vi "Gas Flow 2.vi"() -> ()   [LabVIEW 2011]
uses:
  GlobalVariables.vi
panel:
  out "TMGa #2 2":string="TMGa #2"
  out "MFC Left 8":string="TMIn #1"
  out "MFC Left 7":string="TMIn #1"
  out "MFC Left 6":string="TMIn #1"
  out "MFC Left 5":string="TMIn #1"
  out "MFC Left 4":string="TMIn #1"
  out "MFC Left 3":string="TMIn #1"
  out "MFC Left 2":string="TMIn #1"
  out "MFC Left":string="TMIn #1"
  out "DMHy":string="DMHy"
  out "TMAl #2":string="TMAl #2"
  out "TMAl #1":string="TMAl #1"
  out "TMGa #2":string="TMGa #2"
  out "TMGa #1":string="TMGa #1"
  out "TMIn #2":string="TMIn #2"
  out "Spare":string="Spare"
  out "TMIn #1":string="TMIn #1"
  out "CCl4":string="CCl4"
  out "DEZn":string="DEZn"
  in  "19":bool caption="49"
  in  "20":bool caption="49"
  in  "29":bool caption="49"
  in  "53":bool caption="49"
  in  "54":bool caption="49"
  in  "55":bool caption="49"
  in  "77":bool caption="49"
  in  "78":bool caption="49"
  in  "79":bool caption="49"
  in  "80":bool caption="49"
  in  "56":bool caption="49"
  in  "81":bool caption="49"
  in  "84":bool caption="49"
  in  "24":bool caption="49"
  in  "24":bool caption="49"
  in  "Flip 91/92":bool
  in  "MFC 55":dbl
  out "MFC 54":dbl
  in  "MFC 53":dbl
  out "MFC 52":dbl
  in  "Flip 33/34":bool
  in  "MFC 51":dbl
  out "MFC 50":dbl
  in  "23":bool caption="49"
  in  "25":bool caption="49"
  in  "MFC 49":dbl
  out "MFC 48":dbl
  in  "26":bool caption="49"
  in  "76":bool caption="49"
  in  "75":bool caption="49"
  in  "66":bool caption="49"
  in  "65":bool caption="49"
  in  "68":bool caption="49"
  in  "67":bool caption="49"
  in  "70":bool caption="49"
  in  "69":bool caption="49"
  in  "72":bool caption="49"
  in  "71":bool caption="49"
  in  "74":bool caption="49"
  in  "73":bool caption="49"
  in  "52":bool caption="49"
  in  "51":bool caption="49"
  in  "34":bool caption="49"
  in  "33":bool caption="49"
  in  "MFC10":dbl
  in  "MFC 45":dbl
  in  "MFC 44":dbl
  in  "MFC 01":dbl
  out "MFC10":dbl
  out "MFC 45":dbl
  out "MFC 44":dbl
  out "MFC 01":dbl
  in  "22":bool caption="49"
  in  "21":bool caption="49"
  in  "22":bool caption="49"
  in  "01":bool caption="49"
  in  "02":bool caption="49"
  in  "02":bool caption="49"
  in  "59":bool caption="49"
  in  "27":bool caption="49"
  in  "30":bool caption="49"
  in  "94":bool caption="49"
  in  "93":bool caption="49"
  in  "?":bool caption="49"
  in  "28":bool caption="49"
  in  "31":bool caption="49"
  in  "95":bool caption="49"
  in  "96":bool caption="49"
  in  "90":bool caption="49"
  in  "92":bool caption="49"
  in  "91":bool caption="49"
  in  "CloseVi?":bool
  in  "Close":bool
  # "19"
  # "20"
  # "71/72"
  # "TO EBARA"
  # "Arsine"
  # "AsH3 1-DD VENT"
  # "32"
  # "21"
  # "H2"
  # "33"
  # "TO TURBO PUMP"
  # "23"
  # "69/70"
  # "22"
  # "AsH3 2-DD VENT"
  # "24"
  # "Si2H6 DD VENT"
  # "34"
  # "67/68"
  # "HYDRIDE GROWTH"
  # "Phosphine"
  # "35"
  # "38"
  # "42"
  # "Si2H6 DD VENT"
  # "HYDRIDE VENT"
  # "?"
  # "36"
  # "TO SHROUD"
  # "39"
  # "TO PURGE"
  # "41"
  # "N2"
  # "41"
  # "57"
  # "TO GLOVE BOX"
  # "28"
  # "ALKYL GROWTH"
  # "ALKYL VENT"
  # "27"
  # "ALKYL DD VENT"
  # "57"
  # "28"
  # "27"
  # "VACUUM"
  # "VENT"
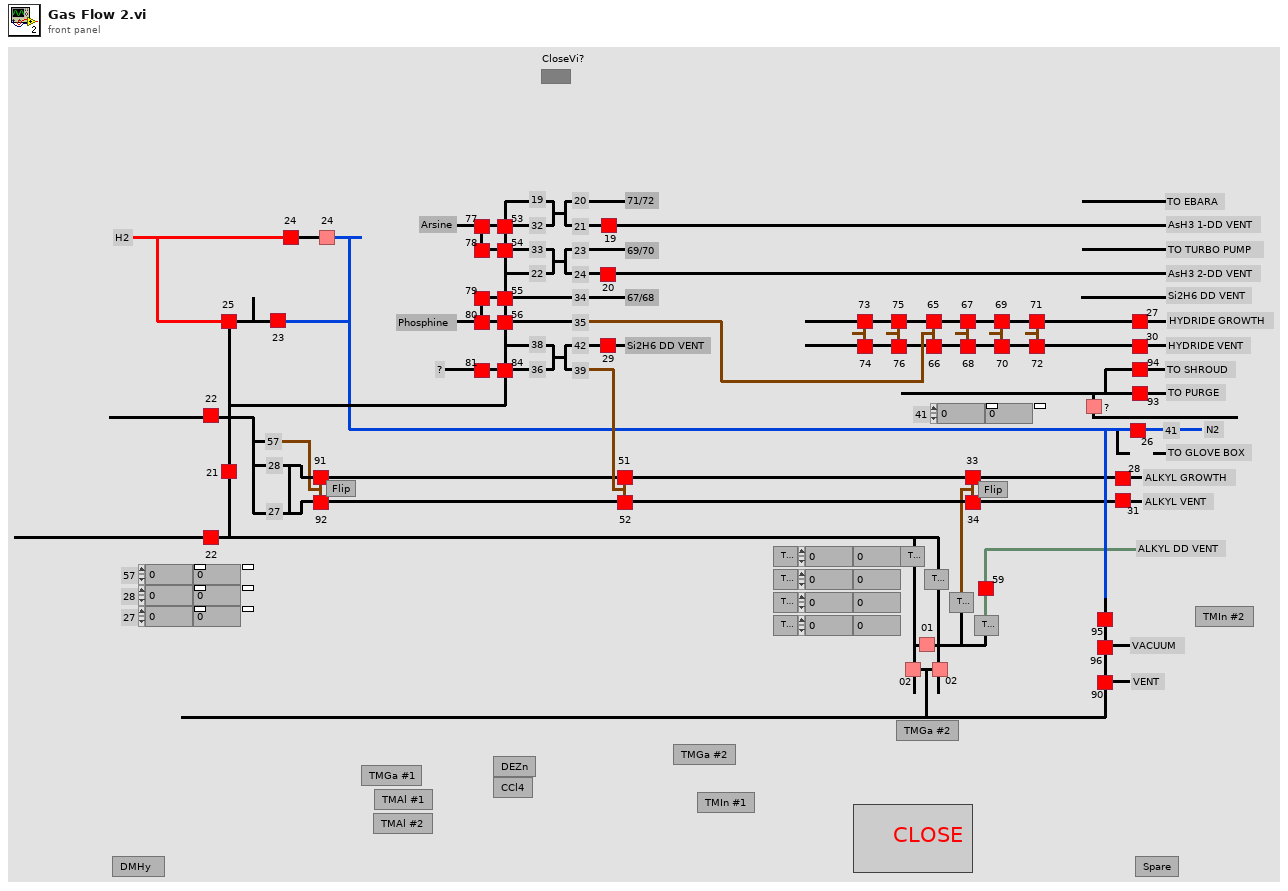
[diagram p1: front panel]
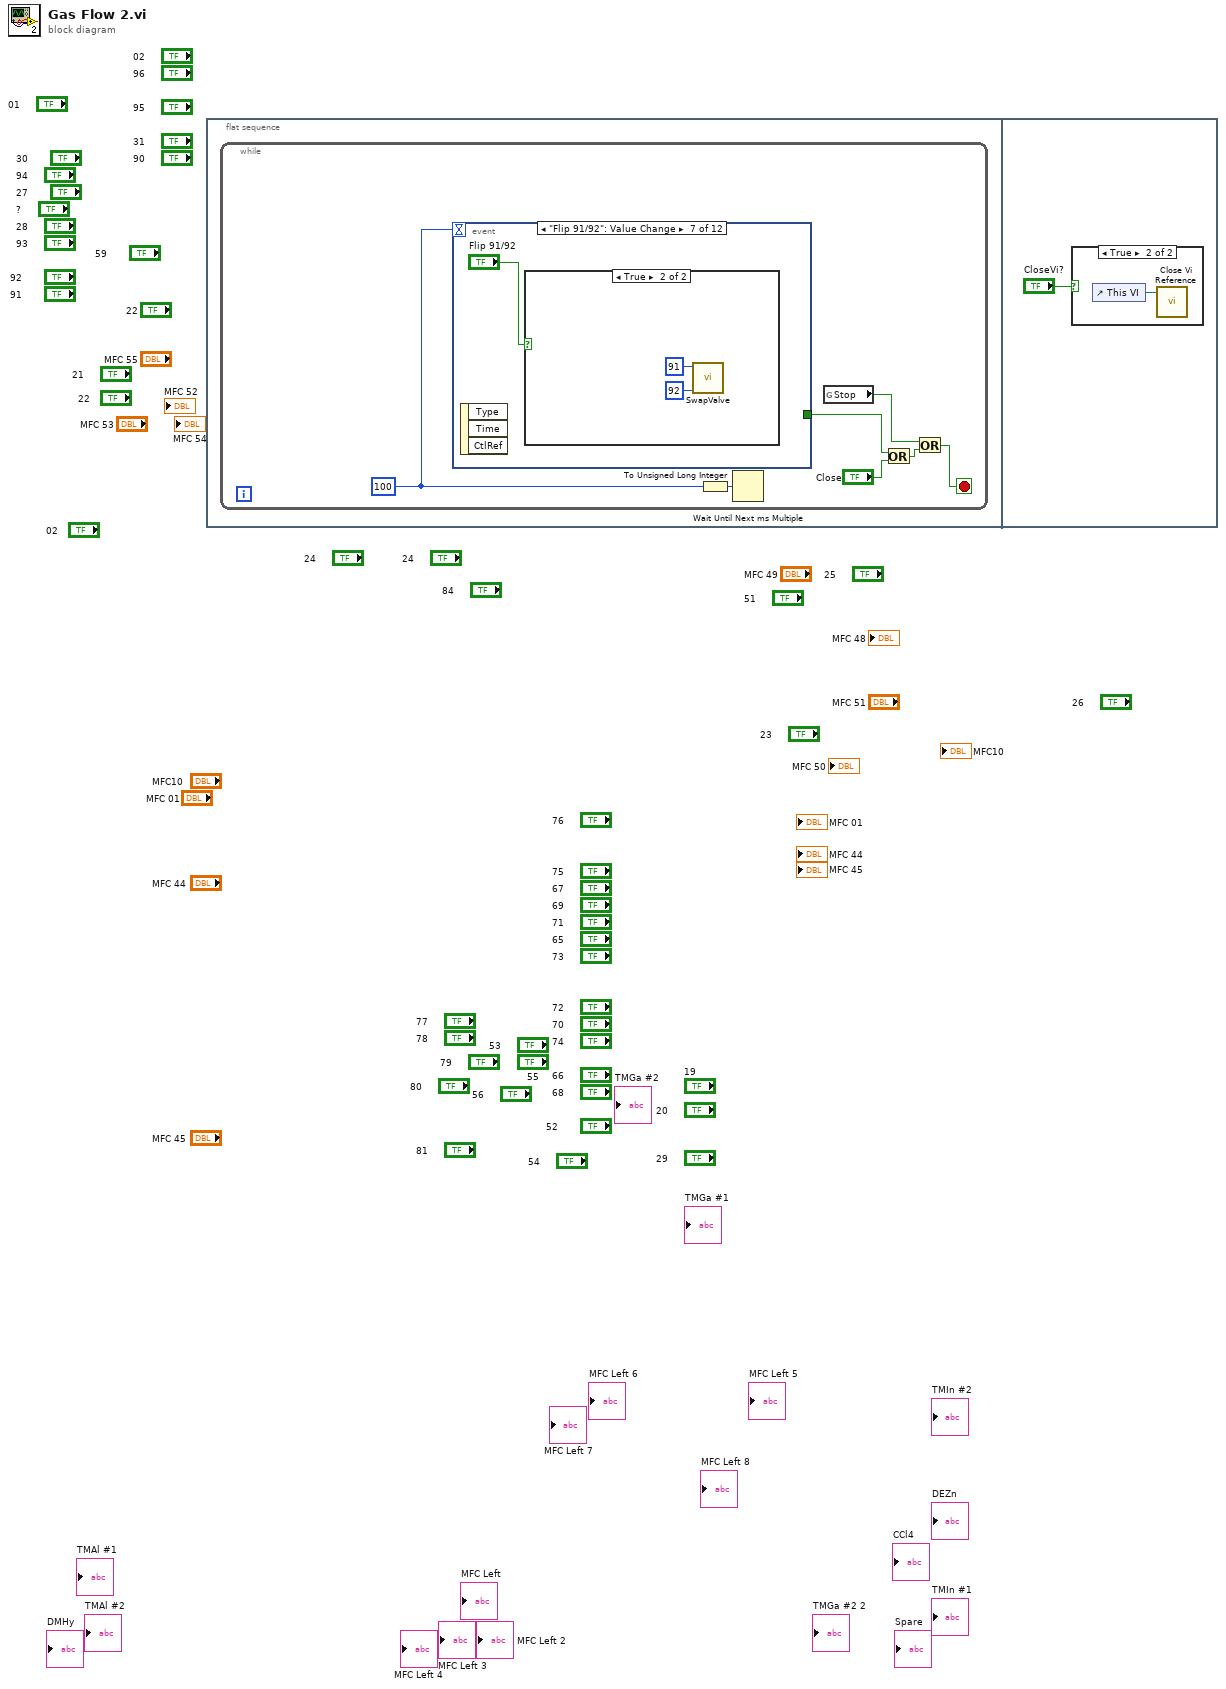
[diagram p0: block diagram]
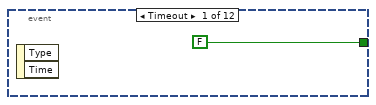
[diagram p2: hidden frame]
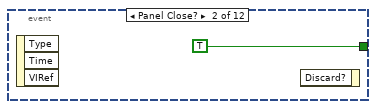
[diagram p3: hidden frame]
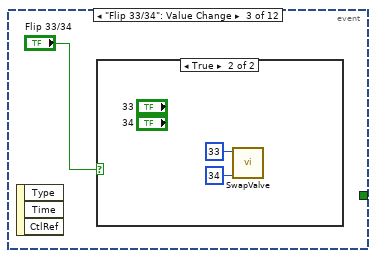
[diagram p4: hidden frame]
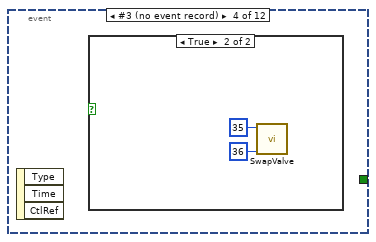
[diagram p6: hidden frame]
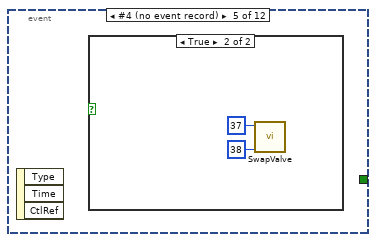
[diagram p8: hidden frame]
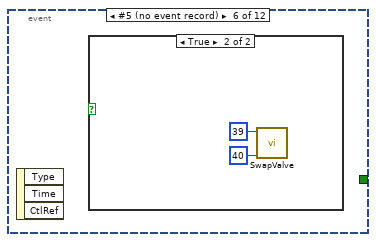
[diagram p10: hidden frame]
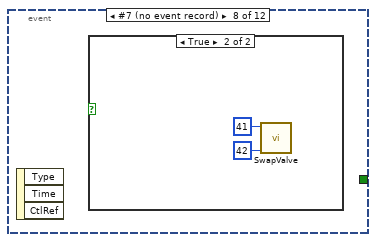
[diagram p13: hidden frame]
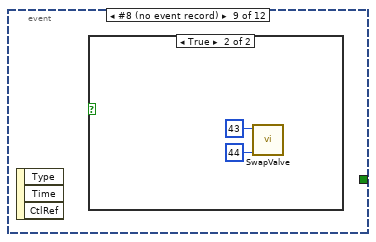
[diagram p15: hidden frame]
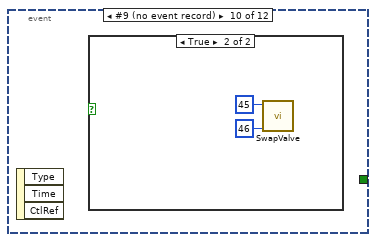
[diagram p17: hidden frame]
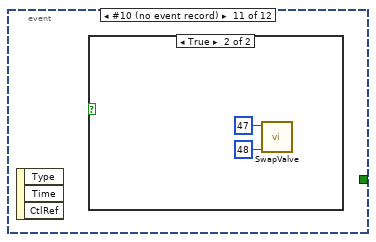
[diagram p19: hidden frame]
diagram:
  n1 = flat-sequence {
    frame #0 {
      n2 = while {
        stop <- w1 stop-if-true
        w2 = 100
        n3 = event shown="[6] \"Flip 91/92\": Value Change" {
          selector: _ -> [_ _ _ _ _ _ _ _ _ _ _ _]
          dyn-events: _ -> [_ _ _ _ _ _ _ _ _ _ _ _]
          timeout: w2 -> [_ _ _ _ _ _ _ _ _ _ _ _]
          tunnel: [FALSE ("y") TRUE ("y") _ _ _ _ _ _ _ _ _ _] -> w4
          event Timeout {
            n4 = event-data() -> ()  [unwired: 1 in, 2 out]
          }
          event Panel Close? {
            n5 = event-data() -> ()  [unwired: 1 in, 3 out]
            n6 = event-data() -> ()  [unwired: 2 in, 1 out]
          }
          event "Flip 33/34": Value Change {
            n7 = event-data() -> ()  [unwired: 1 in, 3 out]
            n8 = case shown="True" "Flip 33/34" {
              frame False {
              }
              frame True {
                n9 = call "SwapValve.vi"("Valve 2"=34, "Valve 1"=33) -> ()  [unwired: 10 in]
              }
            }
          }
          event #3 (no event record) {
            n10 = event-data() -> ()  [unwired: 1 in, 3 out]
            n11 = case shown="True" w13 {
              frame False {
              }
              frame True {
                n12 = call "SwapValve.vi"("Valve 2"=36, "Valve 1"=35) -> ()  [unwired: 10 in]
              }
            }
          }
          event #4 (no event record) {
            n13 = event-data() -> ()  [unwired: 1 in, 3 out]
            n14 = case shown="True" w16 {
              frame False {
              }
              frame True {
                n15 = call "SwapValve.vi"("Valve 2"=38, "Valve 1"=37) -> ()  [unwired: 10 in]
              }
            }
          }
          event #5 (no event record) {
            n16 = event-data() -> ()  [unwired: 1 in, 3 out]
            n17 = case shown="True" w19 {
              frame False {
              }
              frame True {
                n18 = call "SwapValve.vi"("Valve 2"=40, "Valve 1"=39) -> ()  [unwired: 10 in]
              }
            }
          }
          event "Flip 91/92": Value Change {
            n19 = event-data() -> ()  [unwired: 1 in, 3 out]
            n20 = case shown="True" "Flip 91/92" {
              frame False {
              }
              frame True {
                n21 = call "SwapValve.vi"("Valve 2"=92, "Valve 1"=91) -> ()  [unwired: 10 in]
              }
            }
          }
          event #7 (no event record) {
            n22 = event-data() -> ()  [unwired: 1 in, 3 out]
            n23 = case shown="True" w25 {
              frame False {
              }
              frame True {
                n24 = call "SwapValve.vi"("Valve 2"=42, "Valve 1"=41) -> ()  [unwired: 10 in]
              }
            }
          }
          event #8 (no event record) {
            n25 = event-data() -> ()  [unwired: 1 in, 3 out]
            n26 = case shown="True" w28 {
              frame False {
              }
              frame True {
                n27 = call "SwapValve.vi"("Valve 2"=44, "Valve 1"=43) -> ()  [unwired: 10 in]
              }
            }
          }
          event #9 (no event record) {
            n28 = event-data() -> ()  [unwired: 1 in, 3 out]
            n29 = case shown="True" w31 {
              frame False {
              }
              frame True {
                n30 = call "SwapValve.vi"("Valve 2"=46, "Valve 1"=45) -> ()  [unwired: 10 in]
              }
            }
          }
          event #10 (no event record) {
            n31 = event-data() -> ()  [unwired: 1 in, 3 out]
            n32 = case shown="True" w34 {
              frame False {
              }
              frame True {
                n33 = call "SwapValve.vi"("Valve 2"=48, "Valve 1"=47) -> ()  [unwired: 10 in]
              }
            }
          }
          event #11 (no event record) {
            n34 = event-data() -> ()  [unwired: 1 in, 3 out]
            n35 = case shown="True" w37 {
              frame False {
              }
              frame True {
                n36 = call "SwapValve.vi"("Valve 2"=50, "Valve 1"=49) -> ()  [unwired: 10 in]
              }
            }
          }
        }
        n37 = To Unsigned Long Integer(number=w2) -> (unsigned 32bit integer=w3:u32)
        n38 = Wait Until Next ms Multiple(millisecond multiple=w3) -> ()  [unwired: 1 out]
        n39 = global read "GlobalVariables.vi" "Stop"() -> (w7:bool)
        n40 = Or(x=w4, y="Close") -> (x .or. y?=w6:bool)
        n41 = Or(x=w7, y=w6) -> (x .or. y?=w1:bool)
      }
    }
    frame #1 {
      n42 = case shown="True" "CloseVi?" {
        frame False {
        }
        frame True {
          n43 = control-ref of="This VI"() -> (w41:refnum<vi>)
          n44 = call "Close Vi Reference.vi"("reference"=w41) -> ()  [unwired: 9 in, 2 out]
        }
      }
    }
  }
